vi "MG17DebugScript.vi"() -> ()   [LabVIEW 2016]
panel:
  in  "Decrement":bool
  out "Numeric":i32
  out "MG17 Error":errorcluster
  in  "stop":bool
  in  "MG17Motor":refnum<k7>(container)
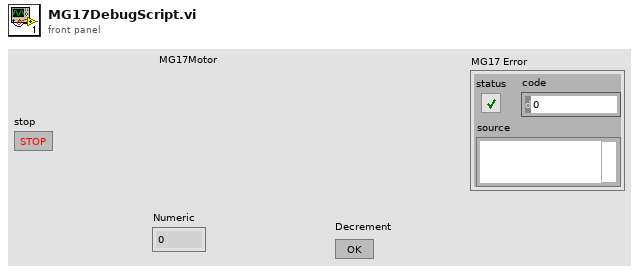
[diagram p1: front panel]
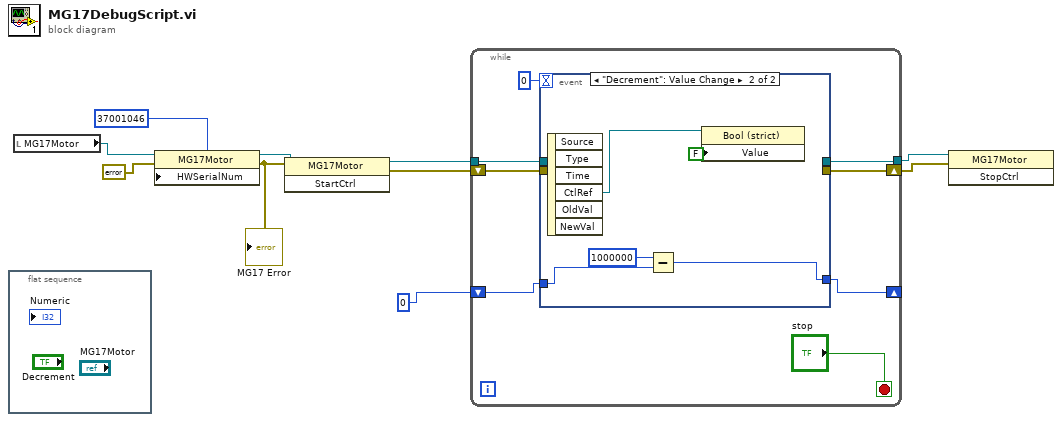
[diagram p0: block diagram]
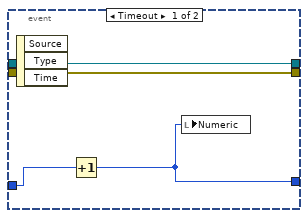
[diagram p2: hidden frame]
diagram:
  n1 = flat-sequence {
    frame #0 {
    }
  }
  n2 = local read "MG17Motor"() -> (w1:refnum<k7>)
  n3 = property class="MG17Motor"(reference=w1, error in=errorcluster {"status"=FALSE, "code"=0, "source"=""} ("error in (no error)"), "HWSerialNum"=37001046) -> (reference out=w9:refnum<k7>, error out=w8:errorcluster)
  "MG17 Error" <- w8
  n4 = invoke class="MG17Motor" method="StartCtrl"(reference=w9, error in=w8) -> (reference out=w6:refnum<k7>, error out=w5:errorcluster)  [unwired: 1 in, 1 out]
  n5 = while {
    tunnel: w6 -> [w16]
    tunnel: [w15] -> w4
    shift-right: [w13] -> w3
    shift-left: w5 -> [w14]
    shift-right: [w11] -> _
    shift-left: 0 -> [w12]
    stop <- "stop" stop-if-true
    n6 = event shown="[1] \"Decrement\": Value Change" {
      selector: _ -> [_ _]
      dyn-events: _ -> [_ _]
      timeout: 0 -> [_ _]
      tunnel: w16 -> [w22 _]
      tunnel: [w22 _] -> w15
      tunnel: w14 -> [w21 _]
      tunnel: [w21 _] -> w13
      tunnel: w12 -> [w20 w27]
      tunnel: [w19 w25] -> w11
      event Timeout {
        n7 = event-data() -> ()  [unwired: 1 in, 3 out]
        n8 = Increment(x=w20) -> (x+1=w19:i32)
        n9 = local write "Numeric"(w19) -> ()
      }
      event "Decrement": Value Change {
        n10 = event-data() -> ("CtlRef"=w24:refnum<vi>)  [unwired: 1 in, 5 out]
        n11 = Subtract(x=1000000, y=w27) -> (x-y=w25:i32)
        n12 = property class="Bool (strict)"(reference=w24, "Value"=FALSE) -> ()  [unwired: 1 in, 2 out]
      }
    }
  }
  n13 = invoke class="MG17Motor" method="StopCtrl"(reference=w4, error in=w3) -> ()  [unwired: 1 in, 3 out]
